vi "Compare without Timestamp.vi"(10 "Status_IED gold":T1, 11 "IED_Status test":T1) -> (3 "Boolean":bool)   [LabVIEW 2018, in "IED Test Framework.lvlib" / "IED Test.lvclass"]
uses:
  IED Test.lvclass
  <vilib>/ORNL/CSEISMIC DDS/CSEISMIC DDS Base/Data Types/IED_Status.ctl
  <vilib>/ORNL/CSEISMIC DDS/CSEISMIC DDS Base/Data Types/Controls/DeviceID.ctl
  <vilib>/ORNL/CSEISMIC DDS/CSEISMIC DDS Base/Data Types/Controls/Timestamp.ctl
  <vilib>/ORNL/CSEISMIC DDS/CSEISMIC DDS Base/CSEISMIC DDS.lvclass
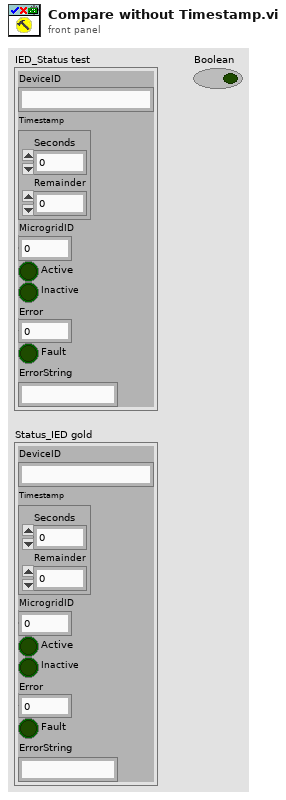
[diagram p1: front panel]
types:
  T1 = typedef "CSEISMIC DDS.lvlib/CSEISMIC DDS.lvclass/IED_Status.ctl" = cluster{"DeviceID":T2, "Timestamp":T3, "MicrogridID":u8, "Active":bool, "Inactive":bool, "Error":i32, "Fault":bool, "ErrorString":string}
  T2 = typedef "CSEISMIC DDS.lvlib/CSEISMIC DDS.lvclass/DeviceID.ctl" = string
  T3 = typedef "CSEISMIC DDS.lvlib/CSEISMIC DDS.lvclass/Timestamp.ctl" = cluster{"Seconds":u64, "Remainder":u64}
  T4 = cluster{"DeviceID":T2, "MicrogridID":u8, "Active":bool, "Inactive":bool, "Error":i32, "Fault":bool, "ErrorString":string}
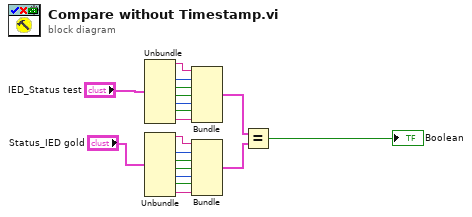
[diagram p0: block diagram]
diagram:
  n1 = Unbundle("IED_Status test") -> ("DeviceID"=w11:T2, "MicrogridID"=w12:u8, "Active"=w13:bool, "Inactive"=w14:bool, "Error"=w15:i32, "Fault"=w16:bool, "ErrorString"=w17:string)  [unwired: 1 out]
  n2 = Unbundle("Status_IED gold") -> ("DeviceID"=w10:T2, "MicrogridID"=w9:u8, "Active"=w8:bool, "Inactive"=w7:bool, "Error"=w6:i32, "Fault"=w5:bool, "ErrorString"=w4:string)  [unwired: 1 out]
  n3 = Bundle("DeviceID"=w11, "MicrogridID"=w12, "Active"=w13, "Inactive"=w14, "Error"=w15, "Fault"=w16, "ErrorString"=w17) -> (w1:T4)  [unwired: 1 in]
  n4 = Bundle("DeviceID"=w10, "MicrogridID"=w9, "Active"=w8, "Inactive"=w7, "Error"=w6, "Fault"=w5, "ErrorString"=w4) -> (w2:T4)  [unwired: 1 in]
  n5 = Equal?(x=w1, y=w2) -> (x = y?=→"Boolean":bool)
